vi "子VI-缺陷长宽比筛选.vi"(9 "判定为筋条的长宽比阈值":i32, 11 "分层测量结果":dbl[][](array[numeric])) -> (2 "初始化的数组":dbl[][](array[numeric]))   [LabVIEW 2018]
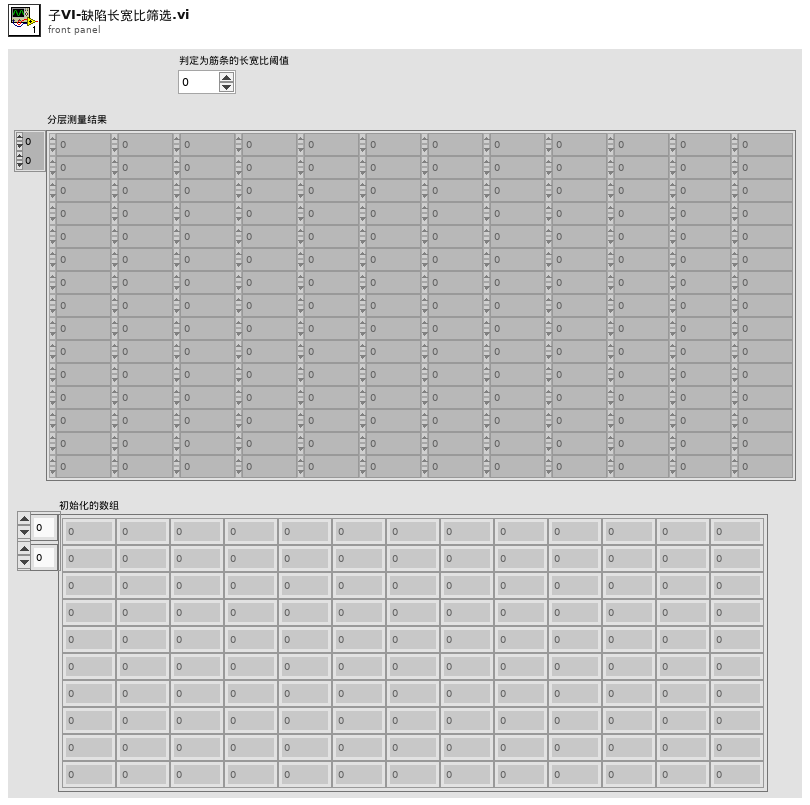
[diagram p1: front panel]
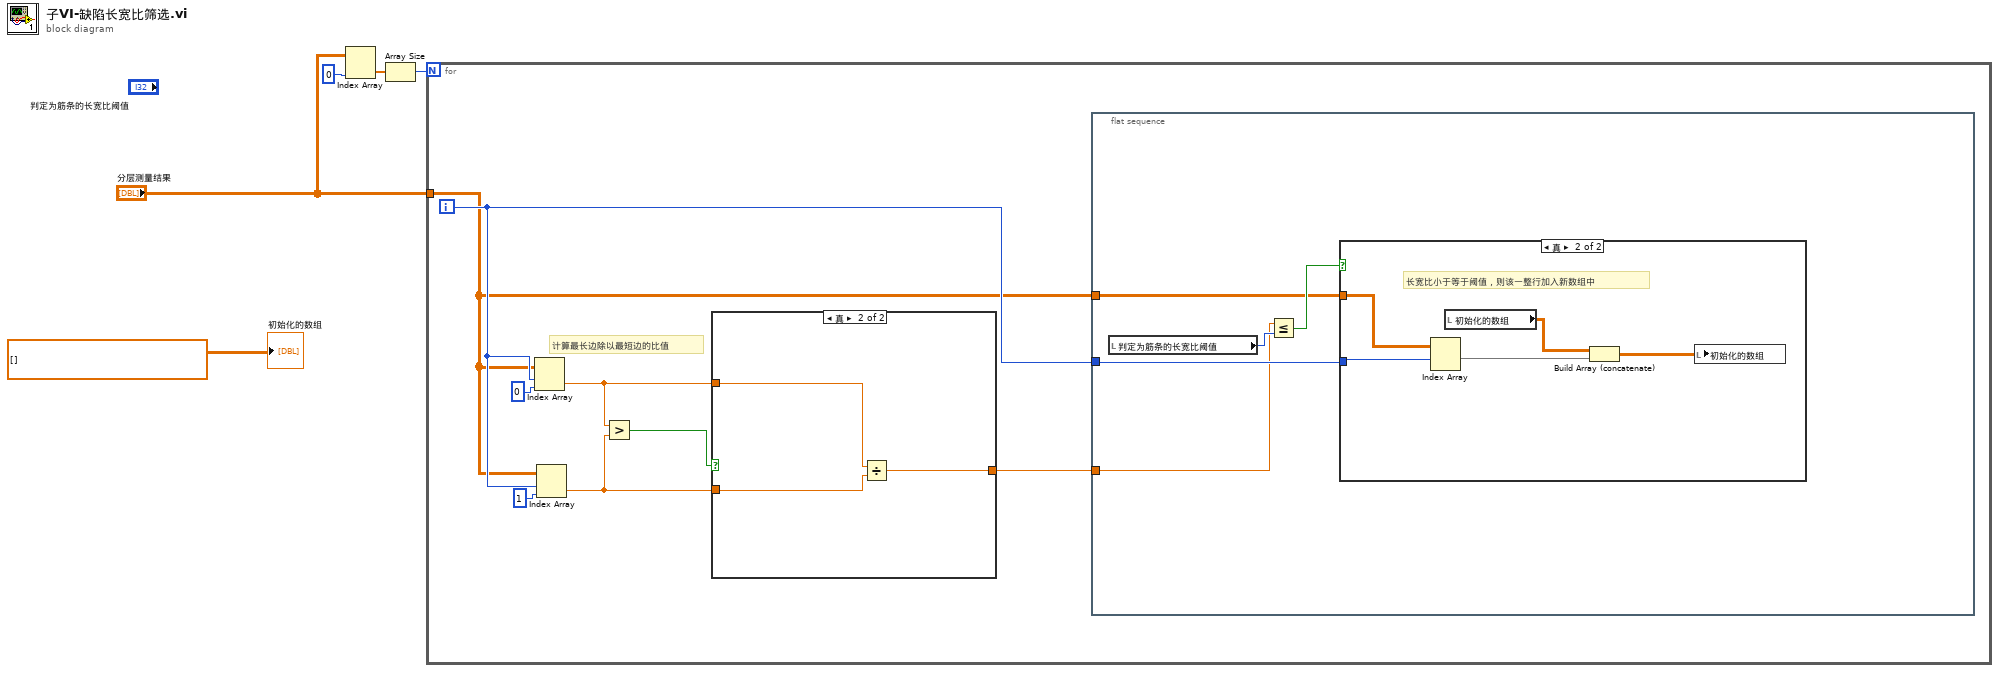
[diagram p0: block diagram]
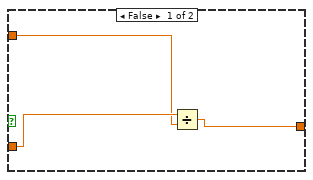
[diagram p3: hidden frame]
diagram:
  n1 = Index Array(array="分层测量结果", index (col)=0 ("禁用的索引 (列)")) -> (element=w3:dbl[])  [unwired: 1 in]
  n2 = Array Size(array=w3) -> (size(s)=w4:i32)
  n3 = for {
    N: w4 -> [_]
    tunnel: "分层测量结果" -> [w7]
    i -> [w8]
    # "计算最长边除以最短边的比值"
    n4 = Index Array(array=w7, index (row)=w8, index (col)=0 ("索引 (列)")) -> (element=w10:dbl)
    n5 = Index Array(array=w7, index (row)=w8, index (col)=1 ("索引 (列)")) -> (element=w9:dbl)
    n6 = Greater?(x=w10, y=w9) -> (0:w11:bool)
    n7 = case shown="真" w11 {
      tunnel: w10 -> [w25 w29]
      tunnel: w9 -> [w26 w28]
      tunnel: [w24 w27] -> w6
      frame False {
        n8 = Divide(x=w26, y=w25) -> (x/y=w24:dbl)
      }
      frame True {
        n9 = Divide(x=w29, y=w28) -> (x/y=w27:dbl)
      }
    }
    n10 = flat-sequence {
      tunnel: w8 -> [w16]
      tunnel: w7 -> [w15]
      tunnel: w6 -> [w14]
      frame #0 {
        n11 = local read "判定为筋条的长宽比阈值"() -> (w17:i32)
        n12 = Less Or Equal?(x=w14, y=w17) -> (x <= y?=w18:bool)
        n13 = case shown="真" w18 {
          tunnel: w16 -> [_ w19]
          tunnel: w15 -> [_ w23]
          frame False {
          }
          frame True {
            # "长宽比小于等于阈值，则该一整行加入新数组中"
            n14 = Index Array(array=w23, index (row)=w19) -> (element=w22:dbl[])  [unwired: 1 in]
            n15 = local read "初始化的数组"() -> (w21:dbl[][])
            n16 = Build Array (concatenate)(w21, w22) -> (w20:dbl[][])
            n17 = local write "初始化的数组"(w20) -> ()
          }
        }
      }
    }
  }
  "初始化的数组" <- dbl[][] [] ("初始化的数组")
